vi "Evaluate Dwell Limits.vi"(8 "Voltage Dwell Count":u32, 9 "Stage Dwell Limit":u16, 10 "Event Count":u16, 11 "Event Dwell Limit":u16) -> (0 "At Stage Dwell Limit?":bool, 1 "Above Stage Dwell Limit?":bool, 3 "Above Event Dwell Limit?":bool)   [LabVIEW 2015]
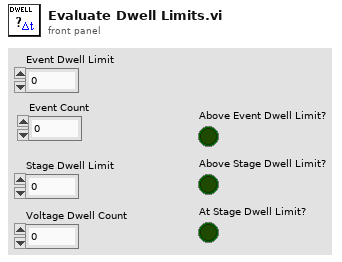
[diagram p1: front panel]
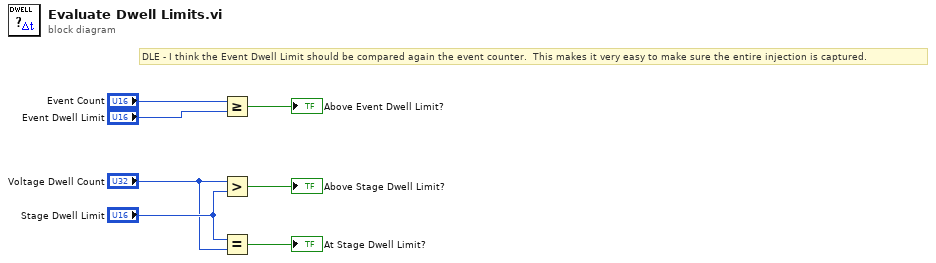
[diagram p0: block diagram]
diagram:
  # "DLE - I think the Event Dwell Limit should be compared again the event counter.  This makes it very easy to make sure the entire injection is captured."
  n1 = Greater Or Equal?(x="Event Count", y="Event Dwell Limit") -> (x >= y?=→"Above Event Dwell Limit?":bool)
  n2 = Greater?(x="Voltage Dwell Count", y="Stage Dwell Limit") -> (0:→"Above Stage Dwell Limit?":bool)
  n3 = Equal?(x="Stage Dwell Limit", y="Voltage Dwell Count") -> (x = y?=→"At Stage Dwell Limit?":bool)
